vi "sweep_dc.vi"(10 "Cluster 4":T4={"numero di sweep ripetute\n(piramidi per dual sweep)"=3, "Delay Time (S)"=0.001, "Numero di punti"=11, "nplc"=0.1, "dual sweep"=FALSE, "autorange source gate"=FALSE, "source_range_gate"=20.0, "String"="1,2,3", "limit-gate"=1.0, "Source Function Gate"=1, "Range Mode Gate"=0, "range-gate"=0.01, "Autozero Mode Gate"=1, "autorange source drain"=FALSE, "source_range_drain"=2.0, "Pulse Start Level (0 V) 2"=-5.0, "Pulse Stop Level (1 V) 2"=1.0, "limit-drain"=1.0, "Source Function Drain"=1, "Range Mode Drain"=0, "range-drain"=0.01, "Autozero Mode Drain"=1, "inverti smu"=FALSE} {"Autozero Mode Drain" items=["Autozero Off", "Autozero Once", "Autozero Auto"]; "range-drain" items=["100 nA"=1e-07, "1 uA"=1e-06, "10 uA"=1e-05, "100 uA"=0.0001, "1 mA"=0.001, "10 mA"=0.01, "100 mA"=0.1, "1 A"=1.0]; "Range Mode Drain" items=["Auto Range Off", "Auto Range On", "Auto Range Follow Limit"]; "Source Function Drain" items=["Current", "Voltage"]; "limit-drain" format="%#_13g"; "source_range_drain" items=["200 mV"=0.2, "2 V"=2.0, "20 V"=20.0, "200 V"=200.0]; "Autozero Mode Gate" items=["Autozero Off", "Autozero Once", "Autozero Auto"]; "range-gate" items=["100 nA"=1e-07, "1 uA"=1e-06, "10 uA"=1e-05, "100 uA"=0.0001, "1 mA"=0.001, "10 mA"=0.01, "100 mA"=0.1, "1 A"=1.0]; "Range Mode Gate" items=["Auto Range Off", "Auto Range On", "Auto Range Follow Limit"]; "Source Function Gate" items=["Current", "Voltage"]; "limit-gate" format="%#_13g"; "source_range_gate" items=["200 mV"=0.2, "2 V"=2.0, "20 V"=20.0, "200 V"=200.0]; "nplc" items=["0,01"=0.01, "0,1"=0.1, "1"=1.0]}, 11 "Cluster":T3={"VISA resource name"="USB0::0x05E6::0x2612::4671051::INSTR", "error in (no error)"={"status"=FALSE, "code"=0, "source"=""}}) -> (2 "Cluster 3":T1, 3 "Cluster 2":T2)   [LabVIEW 2026]
uses:
  <instrlib>/Keithley 2600 Series/Keithley 2600 Series.lvlib
panel:
  out "range misurato":string
  out "range misurato 2":string
  out "intervallo tra due misure approx (S)":dbl
  out "Frequenza di rete (Hz)":dbl
  out "finestra di misura (S)":dbl
  # "Impostazioni connessione"
  # "tabella valori"
  # "Impostazioni funzione source"
  # "Impostazioni comuni"
  # "DRAIN"
  # "GATE"
  # "non utilizzato...funzioni di lua per automatizzare il range"
  # "Controllo misura"
  # "Impostazioni funzione misura"
  # "DRAIN"
  # "GATE"
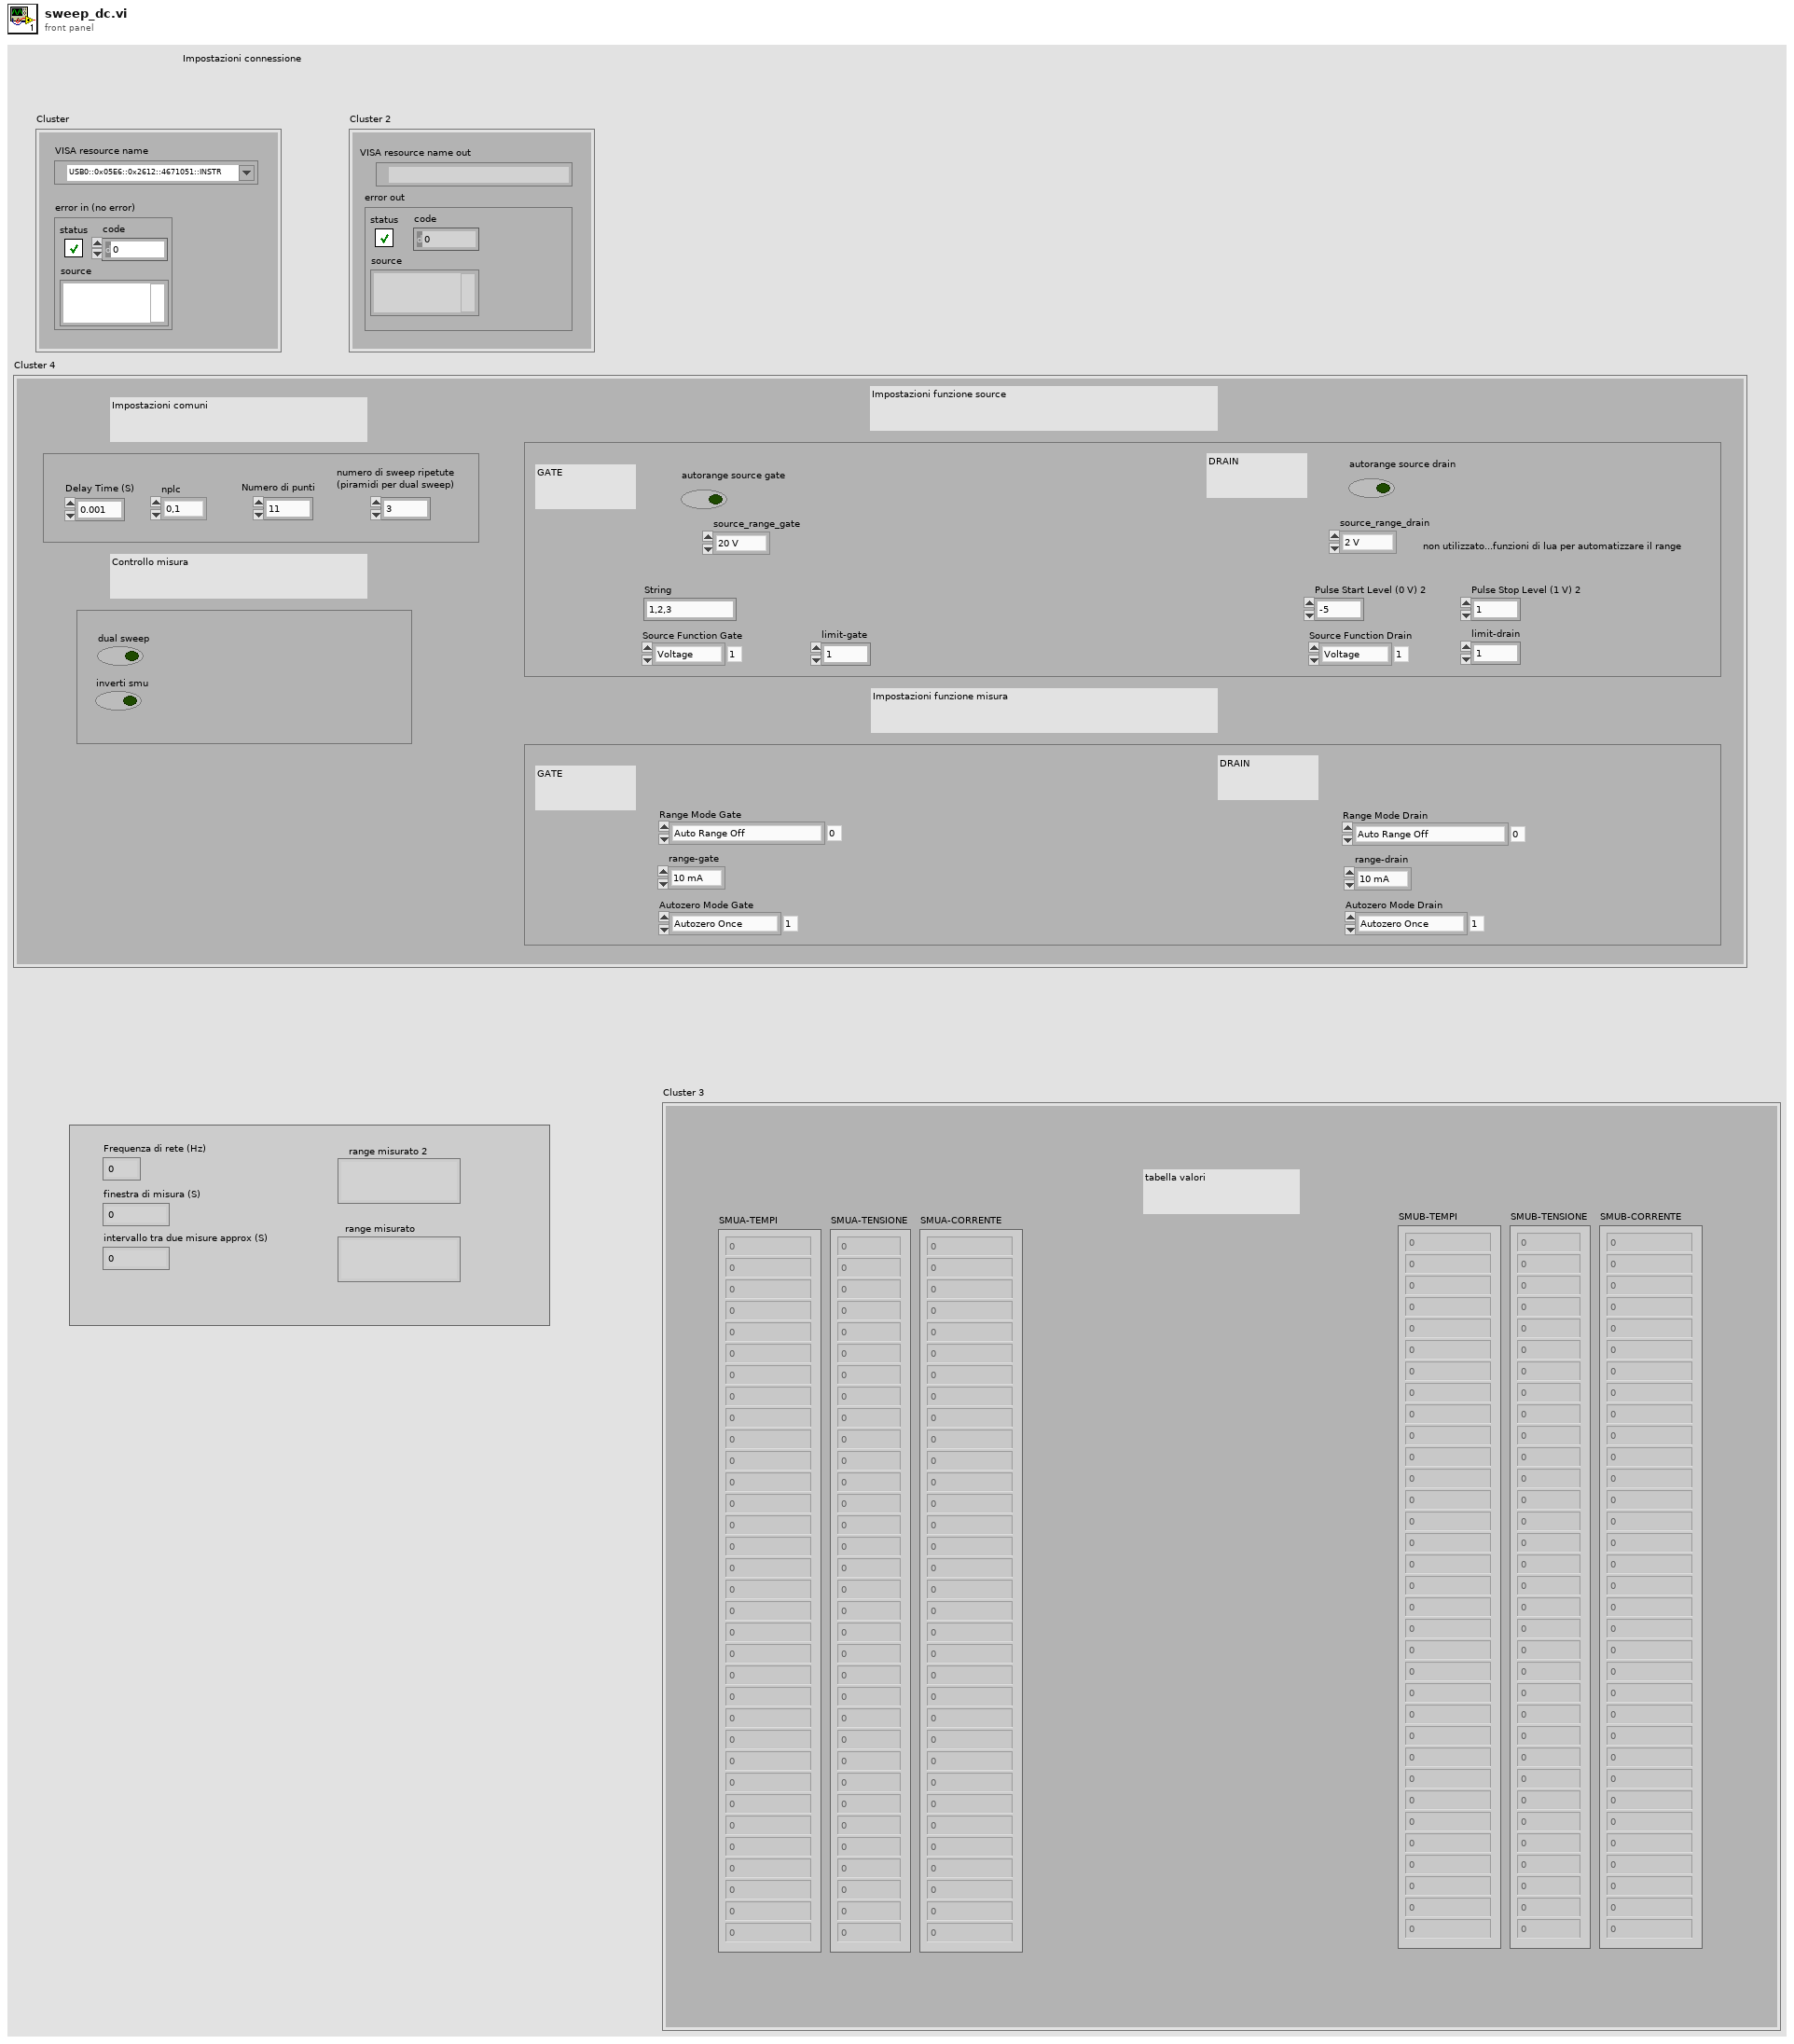
[diagram p1: front panel]
types:
  T1 = cluster{"SMUA-CORRENTE":dbl[], "SMUA-TENSIONE":dbl[], "SMUA-TEMPI":dbl[], "SMUB-CORRENTE":dbl[], "SMUB-TENSIONE":dbl[], "SMUB-TEMPI":dbl[]}
  T2 = cluster{"VISA resource name out":refnum<visa-resource-name>, "error out":errorcluster}
  T3 = cluster{"VISA resource name":refnum<visa-resource-name>, "error in (no error)":errorcluster}
  T4 = cluster{"numero di sweep ripetute\n(piramidi per dual sweep)":i32, "Delay Time (S)":dbl, "Numero di punti":i32, "nplc":dbl, "dual sweep":bool, "autorange source gate":bool, "source_range_gate":dbl, "String":string, "limit-gate":dbl, "Source Function Gate":i32, "Range Mode Gate":i32, "range-gate":dbl, "Autozero Mode Gate":i32, "autorange source drain":bool, "source_range_drain":dbl, "Pulse Start Level (0 V) 2":dbl, "Pulse Stop Level (1 V) 2":dbl, "limit-drain":dbl, "Source Function Drain":i32, "Range Mode Drain":i32, "range-drain":dbl, "Autozero Mode Drain":i32, "inverti smu":bool}
  T5 = cluster{"CORRENTE":dbl[], "TENSIONE":dbl[], "TEMPI":dbl[], "CORRENTE":dbl[], "TENSIONE":dbl[], "TEMPI":dbl[]}
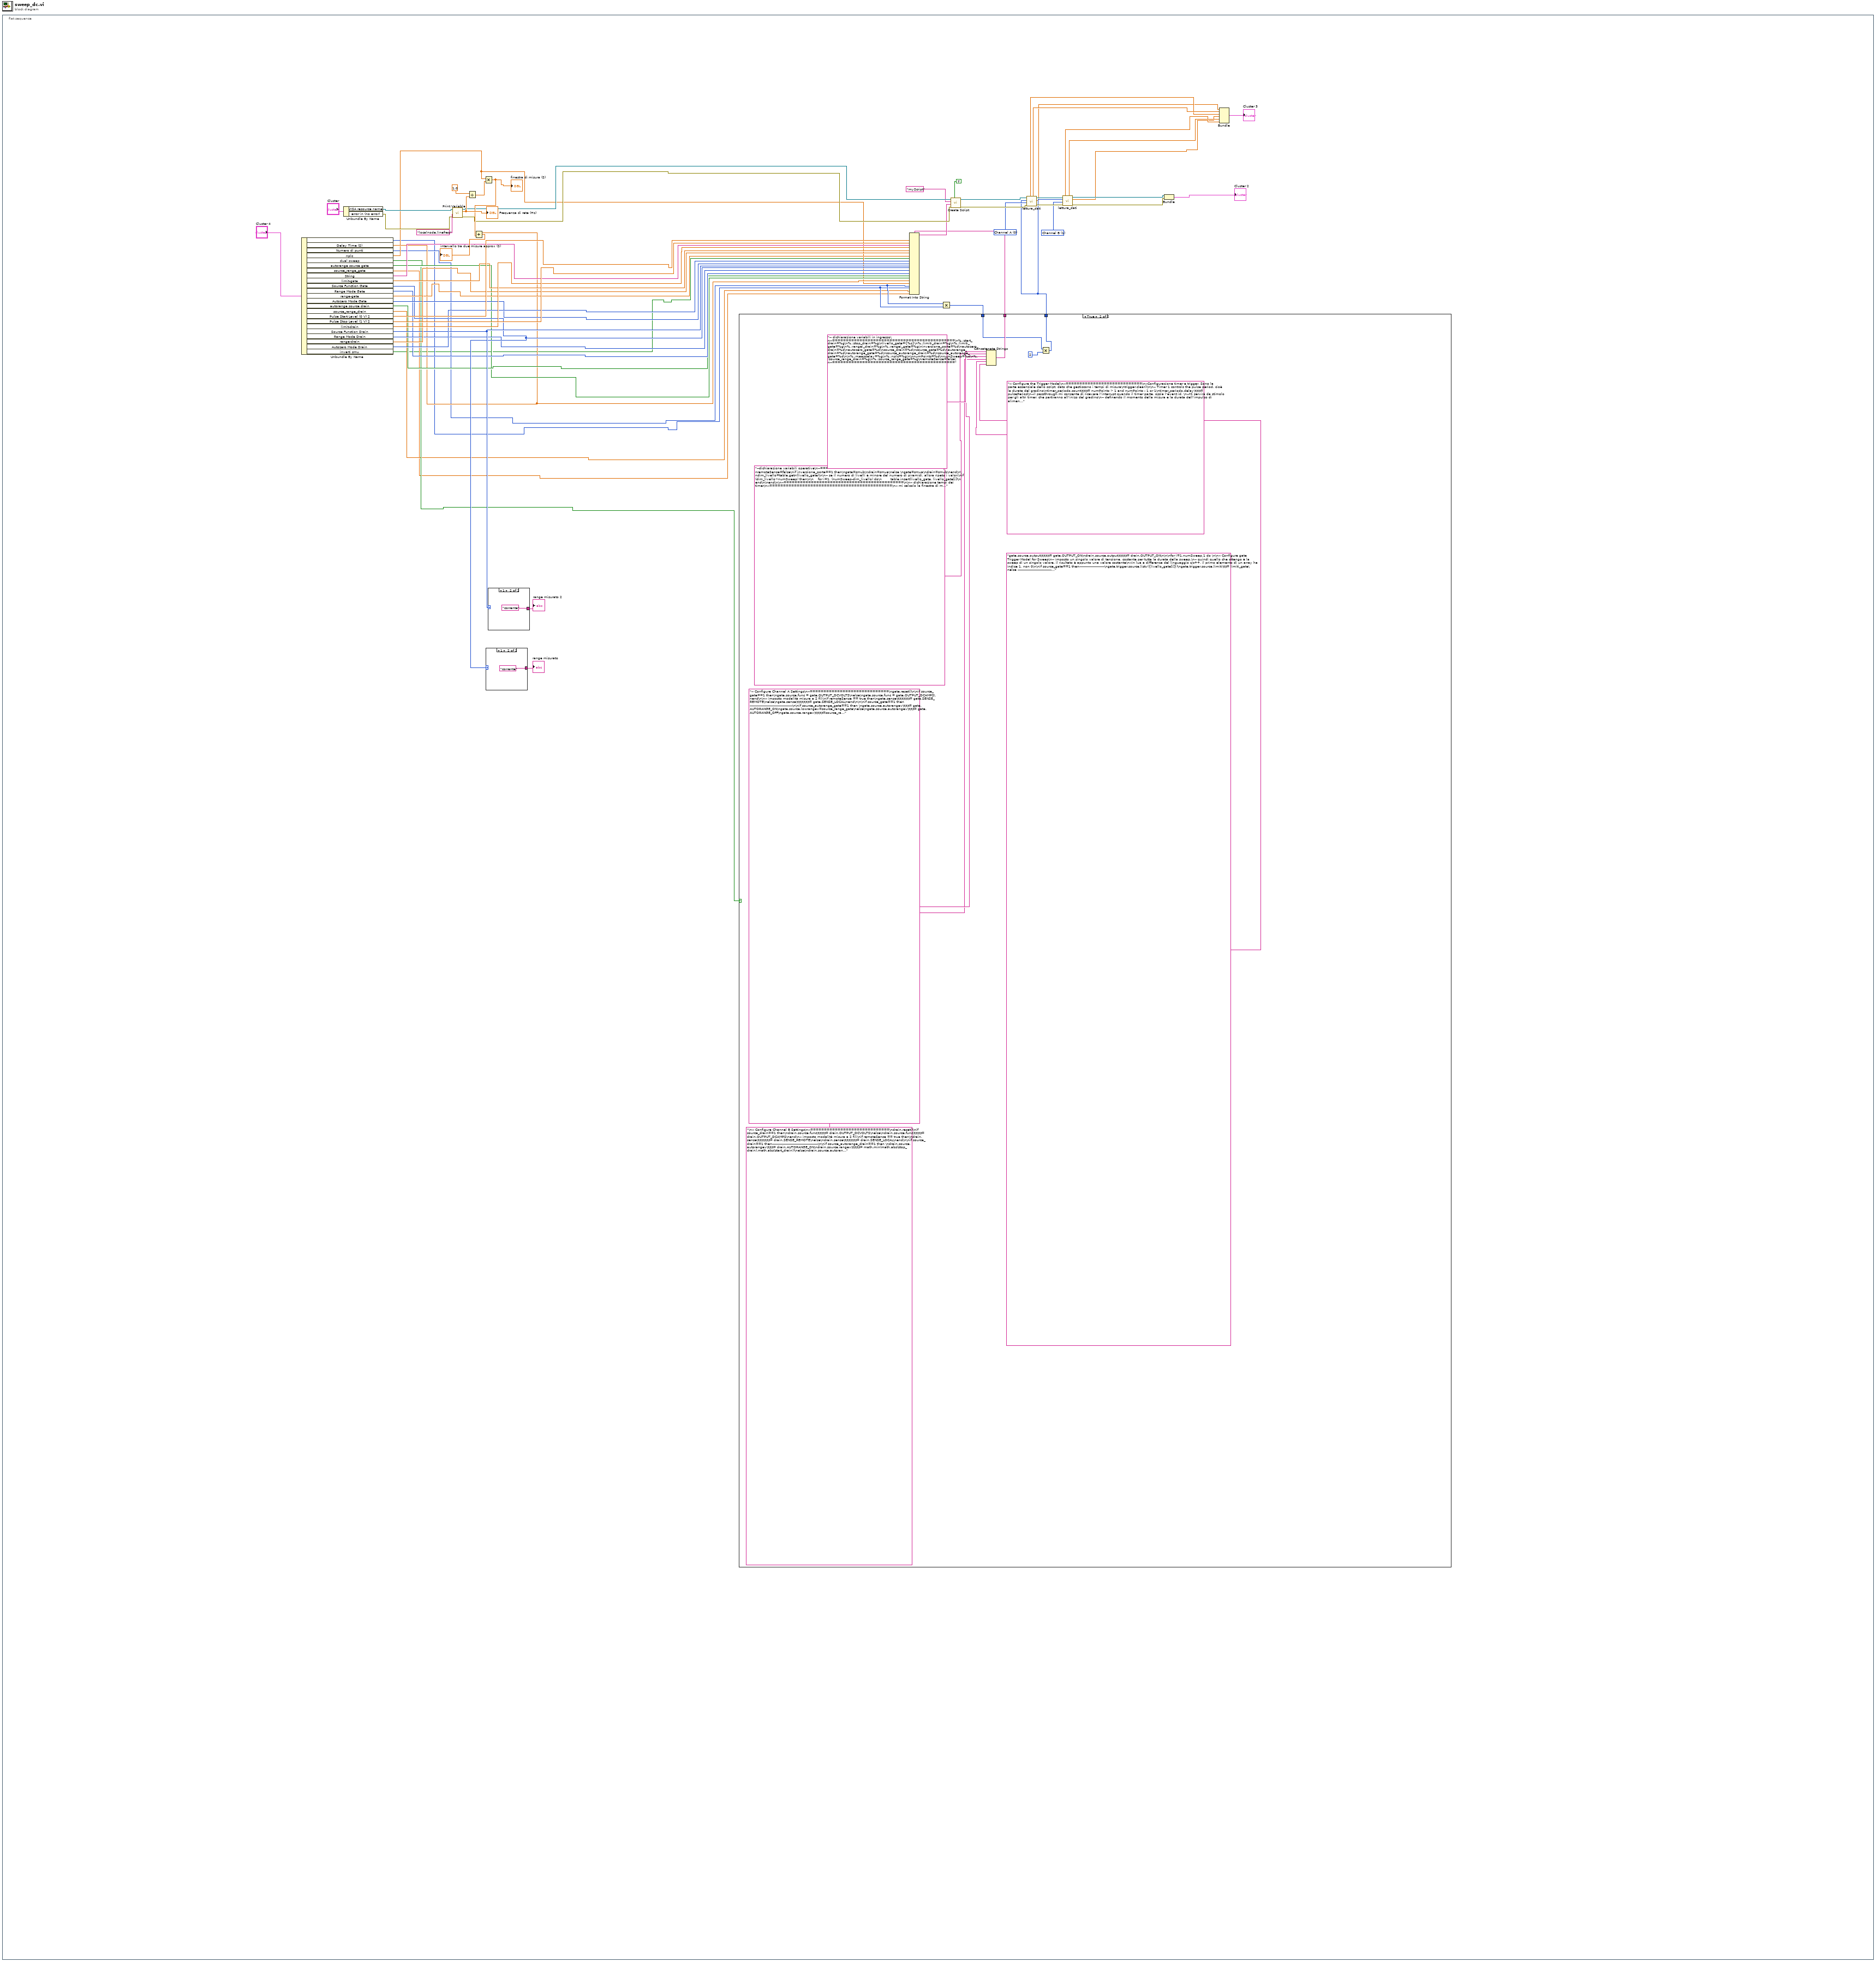
[diagram p0: block diagram]
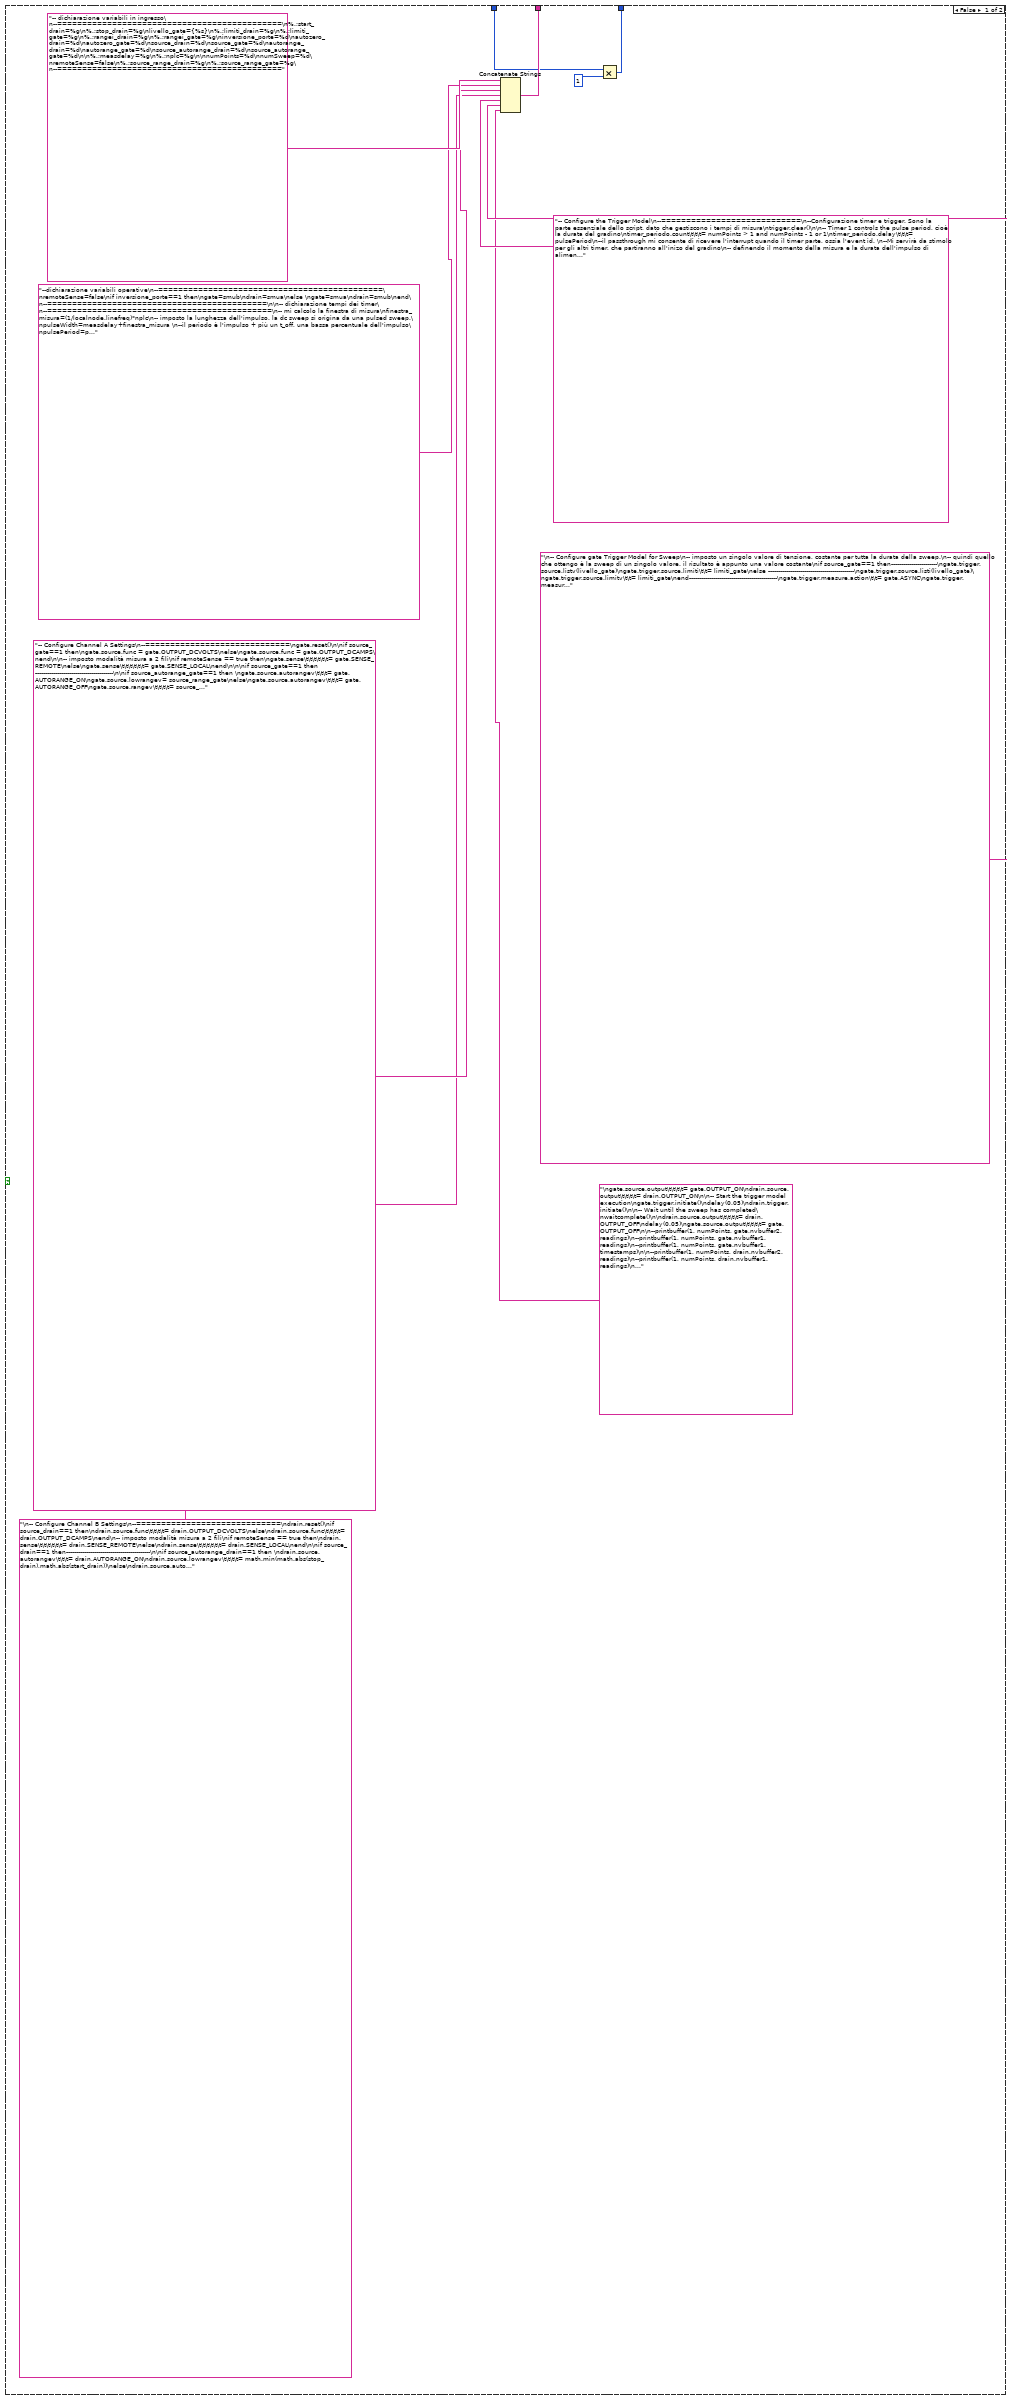
[diagram p2: hidden frame]
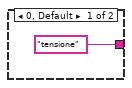
[diagram p3: hidden frame]
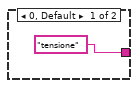
[diagram p4: hidden frame]
diagram:
  n1 = flat-sequence {
    frame #0 {
      w41 = 1 items=["Channel A", "Channel B"] ("Source Measure Unit Channel (0: Channel A)")
      w42 = 0 items=["Channel A", "Channel B"] ("Source Measure Unit Channel (0: Channel A)")
      n2 = Unbundle By Name("Cluster 4") -> ("numero di sweep ripetute\n(piramidi per dual sweep)"=w5:i32, "Delay Time (S)"=w8:dbl, "Numero di punti"=w6:i32, "nplc"=w7:dbl, "dual sweep"=w4:bool, "autorange source gate"=w9:bool, "source_range_gate"=w2:dbl, "String"=w21:string, "limit-gate"=w19:dbl, "Source Function Gate"=w13:i32, "Range Mode Gate"=w11:i32, "range-gate"=w17:dbl, "Autozero Mode Gate"=w15:i32, "autorange source drain"=w10:bool, "source_range_drain"=w3:dbl, "Pulse Start Level (0 V) 2"=w23:dbl, "Pulse Stop Level (1 V) 2"=w22:dbl, "limit-drain"=w20:dbl, "Source Function Drain"=w14:i32, "Range Mode Drain"=w12:i32, "range-drain"=w18:dbl, "Autozero Mode Drain"=w16:i32, "inverti smu"=w1:bool)
      n3 = Unbundle By Name("Cluster") -> ("VISA resource name"=w31:refnum<visa-resource-name>, "error in (no error)"=w30:errorcluster)
      n4 = call <instrlib>:"Print Variable.vi"("error in (no error)"=w30, "Variable Name"="localnode.linefreq", "VISA resource name"=w31) -> ("error out"=w52:errorcluster, "Number"=w56:dbl, "VISA resource name out"=w53:refnum<visa-resource-name>)  [unwired: 5 in, 1 out]
      "Frequenza di rete (Hz)" <- w56
      n5 = Divide(x=1.0, y=w56) -> (x/y=w58:dbl)
      n6 = Multiply(x=w7, y=w58) -> (x*y=w54:dbl)
      "finestra di misura (S)" <- w54
      n7 = Add(x=w8, y=w54) -> (x+y=→"intervallo tra due misure approx (S)":dbl)
      n8 = case shown="1" w13 {
        tunnel: ["tensione" "corrente"] -> w50
        frame 0, Default {
        }
        frame 1 {
        }
      }
      "range misurato" <- w50
      n9 = case shown="1" w14 {
        tunnel: ["tensione" "corrente"] -> w51
        frame 0, Default {
        }
        frame 1 {
        }
      }
      "range misurato 2" <- w51
      n10 = Multiply(x=w6, y=w5) -> (x*y=w39:i32)
      n11 = case shown="True" w4 {
        tunnel: [w63 w74] -> w40
        tunnel: w39 -> [w62 w72]
        tunnel: [w61 w73] -> w38
        frame False {
          n12 = Concatenate Strings("-- dichiarazione variabili in ingresso\n--=============================================\n%.;start_drain=%g\n%.;stop_drain=%g\nlivello_gate={%s}\n%.;limiti_drain=%g\n%.;limiti_gate=%g\n%.;rangei_drain=%g\n%.;rangei_gate=%g\ninversione_porte=%d\nautozero_drain=%d\nautozero_gate=%d\nsource_drain=%d\nsource_gate=%d\nautorange_drain=%d\nautorange_gate=%d\nsource_autorange_drain=%d\nsource_autorange_gate=%d\n\n%.;measdelay=%g\n%.;nplc=%g\n\nnumPoints=%d\nnumSweep=%d\nremoteSense=false\n%.;source_range_drain=%g\n%.;source_range_gate=%g\n--=============================================", "--dichiarazione variabili operative\n--=============================================\nremoteSense=false\nif inversione_porte==1 then\ngate=smub\ndrain=smua\nelse \ngate=smua\ndrain=smub\nend\n--============================================\n\n-- dichiarazione tempi dei timer\n--=============================================\n-- mi calcolo la finestra di misura\nfinestra_misura=(1/localnode.linefreq)*nplc\n-- imposto la lunghezza dell'impulso. la dc sweep si origina da una pulsed sweep.\npulseWidth=measdelay+finestra_misura \n--il periodo è l'impulso + più un t_off, una bassa percentuale dell'impulso\npulsePeriod=pulseWidth+(pulseWidth*1/100) \n\n--=============================================\n\n-- dichiarazione timer e gestore eventi\n--=============================================\n-- Timer 1: timer periodo (larghezza gradino)\ntimer_periodo=trigger.timer[1]\n-- Timer 2: Timer ritardo misura\ntimer_misura=trigger.timer[2]\n-- Timer 3: Pulse Width Timer\ntimer_larghezza_impulso=trigger.timer[3]\n\n-- Gestore eventi 1: Event Blender per la partenza di iniziale di smua e l'aggiornamento di smua al trigger di smub\ngestore_avvio_gate=trigger.blender[1]\n--=============================================", "-- Configure Channel A Settings\n--=============================\ngate.reset()\n\nif source_gate==1 then\ngate.source.func = gate.OUTPUT_DCVOLTS\nelse\ngate.source.func = gate.OUTPUT_DCAMPS\nend\n\n-- imposto modalità misura a 2 fili\nif remoteSense == true then\ngate.sense\t\t\t\t\t\t= gate.SENSE_REMOTE\nelse\ngate.sense\t\t\t\t\t\t= gate.SENSE_LOCAL\nend\n\n\nif source_gate==1 then ---------------------------------------\n\nif source_autorange_gate==1 then \ngate.source.autorangev\t\t\t= gate.AUTORANGE_ON\ngate.source.lowrangev= source_range_gate\nelse\ngate.source.autorangev\t\t\t= gate.AUTORANGE_OFF\ngate.source.rangev\t\t\t\t= source_range_gate\nend \n\ngate.source.levelv\t\t\t\t= 0\n-- Set the DC bias limit.  This is not the limit used during the pulses. ma è il valore di idle della gate\ngate.source.limiti\t\t\t\t= limiti_gate\n\nelse------------------------\n\nif source_autorange_gate==1 then\ngate.source.autorangei\t\t\t= gate.AUTORANGE_ON\ngate.source.lowrangei=source_range_gate\nelse\ngate.source.autorangei\t\t\t= gate.AUTORANGE_OFF\ngate.source.rangei\t\t\t=source_range_gate\nend\n\ngate.source.leveli\t\t\t\t= 0\n-- Set the DC bias limit.  This is not the limit used during the pulses. ma è il valore di idle della gate\ngate.source.limitv\t\t\t\t= limiti_gate\nend --------------------------------------------------\n\n\n-- Disabling Auto-Ranging and Auto-Zero ensures accurate and consistent timing\nif autozero_gate==0 then\ngate.measure.autozero\t\t\t= gate.AUTOZERO_OFF\nelseif autozero_gate==1 then\ngate.measure.autozero\t\t\t= gate.AUTOZERO_ONCE\nelse\ngate.measure.autozero\t\t\t= gate.AUTOZERO_AUTO\nend\n\nif autorange_gate==0 then ------------------------\n\nif source_gate==1 then\ngate.measure.autorangei\t\t\t= gate.AUTORANGE_OFF\ngate.measure.rangei\t\t\t\t= rangei_gate\nelse\ngate.measure.autorangev\t\t\t= gate.AUTORANGE_OFF\ngate.measure.rangev\t\t\t\t= rangei_gate\nend\n\nelseif  autorange_gate==1 then -----------\n\nif source_gate==1 then\ngate.measure.autorangei\t\t\t= gate.AUTORANGE_ON\ngate.measure.lowrangei\t\t\t\t= rangei_gate\nelse\ngate.measure.autorangev\t\t\t= gate.AUTORANGE_ON\ngate.measure.lowrangev\t\t\t\t= rangei_gate\nend\n\nelse --------------------------\n\nend -------------------------------\n\ngate.measure.nplc\t\t\t\t= nplc\n-- A timer will be used to set the measure delay and synchronize the measurement\n-- between the two SMUs so set the built in delay to 0.\ngate.measure.delay\t\t\t\t= 0\n\n-- Prepare the Reading Buffers\ngate.nvbuffer1.clear()\ngate.nvbuffer1.collecttimestamps= 1\ngate.nvbuffer2.clear()\ngate.nvbuffer2.collecttimestamps = 1\n--=============================\n-- End Channel A Settings", "\n-- Configure Channel B Settings\n--=============================\ndrain.reset()\nif source_drain==1 then\ndrain.source.func\t\t\t\t= drain.OUTPUT_DCVOLTS\nelse\ndrain.source.func\t\t\t\t= drain.OUTPUT_DCAMPS\nend\n-- imposto modalità misura a 2 fili\nif remoteSense == true then\ndrain.sense\t\t\t\t\t\t= drain.SENSE_REMOTE\nelse\ndrain.sense\t\t\t\t\t\t= drain.SENSE_LOCAL\nend\n\nif source_drain==1 then------------------------------------------\n\nif source_autorange_drain==1 then \ndrain.source.autorangev\t\t\t= drain.AUTORANGE_ON\ndrain.source.lowrangev\t\t\t\t= math.min(math.abs(stop_drain),math.abs(start_drain))\nelse\ndrain.source.autorangev\t\t\t= drain.AUTORANGE_OFF\ndrain.source.rangev\t\t\t\t=  math.max(math.abs(stop_drain),math.abs(start_drain))\nend\n\ndrain.source.levelv\t\t\t\t= 0\n-- Set the DC bias limit.  This is not the limit used during the pulses. ma è il valore di idle della smu\ndrain.source.limiti\t\t\t\t= limiti_drain\nelse----------------------------------------------------\nif source_autorange_drain==1 then \ndrain.source.autorangei\t\t\t= drain.AUTORANGE_ON\ndrain.source.lowrangei\t\t\t\t= math.min(math.abs(stop_drain),math.abs(start_drain))\nelse\ndrain.source.autorangei\t\t\t= drain.AUTORANGE_OFF\ndrain.source.rangei\t\t\t\t= math.max(math.abs(stop_drain),math.abs(start_drain))\nend\ndrain.source.leveli\t\t\t\t= 0\n-- Set the DC bias limit.  This is not the limit used during the pulses. ma è il valore di idle della smu\ndrain.source.limitv\t\t\t\t= limiti_drain\nend----------------------------------------------\n\n-- Disabling Auto-Ranging and Auto-Zero ensures accurate and consistent timing\n\nif autozero_drain==0 then\ndrain.measure.autozero\t\t\t= drain.AUTOZERO_OFF\nelseif autozero_drain==1 then\ndrain.measure.autozero\t\t\t= drain.AUTOZERO_ONCE\nelseif autozero_drain==2 then\ndrain.measure.autozero\t\t\t= drain.AUTOZERO_AUTO\nend\n\nif autorange_drain==0 then --------------------------------\n\nif source_drain==1 then\ndrain.measure.autorangei\t\t\t= drain.AUTORANGE_OFF\ndrain.measure.rangei\t\t\t\t= rangei_drain\nelse\ndrain.measure.autorangev\t\t\t= drain.AUTORANGE_OFF\ndrain.measure.rangev\t\t\t\t= rangei_drain\nend\n\n\n\nelseif  autorange_drain==1 then ----------------------------\n\nif source_drain==1 then\ndrain.measure.autorangei\t\t\t= drain.AUTORANGE_ON\ndrain.measure.lowrangei\t\t\t\t= rangei_drain\nelse\ndrain.measure.autorangev\t\t\t= drain.AUTORANGE_ON\ndrain.measure.lowrangev\t\t\t\t= rangei_drain\nend\n\nelse\n\nend --------------------------------------------------------------\n\ndrain.measure.nplc\t\t\t\t= nplc\n-- A timer will be used to set the measure delay and synchronize the measurement\n-- between the two SMUs so set the built in delay to 0.\ndrain.measure.delay\t\t\t\t= 0\n\n-- Prepare the Reading Buffers\ndrain.nvbuffer1.clear()\ndrain.nvbuffer1.collecttimestamps= 1\ndrain.nvbuffer2.clear()\ndrain.nvbuffer2.collecttimestamps= 1\n--=============================\n-- End Channel B Settings", "-- Configure the Trigger Model\n--============================\n--Configurazione timer e trigger. Sono la parte essenziale dello script, dato che gestiscono i tempi di misura\ntrigger.clear()\n\n-- Timer 1 controls the pulse period, cioè la durata del gradino\ntimer_periodo.count\t\t\t= numPoints > 1 and numPoints - 1 or 1\ntimer_periodo.delay\t\t\t= pulsePeriod\n--il passthrough mi consente di ricevere l'interrupt quando il timer parte, ossia l'event id. \n--Mi servirà da stimolo per gli altri timer, che partiranno all'inizo del gradino\n-- definendo il momento della misura e la durata dell'impulso di alimentazione\ntimer_periodo.passthrough\t= true\n-- il timer 1 parte quando la drain, in questo caso, inizia la sweep: cioè entra nello stato armed\ntimer_periodo.stimulus\t\t= drain.trigger.ARMED_EVENT_ID \n\n-- Timer 2 controls the measurement. il timer 2 gestisce il ritardo di misura. scaduto quello, inizia la finestra di misura\ntimer_misura.count\t\t\t= 1\ntimer_misura.delay\t\t\t= measdelay\n-- il passthrough è false perchè l'interrupt lo produrre alla fine. \n-- Scaduto il delay di misura, inizia la finestra di misura\ntimer_misura.passthrough\t= false\n--il timer 1 grazie al passthrough mi fa partire il timer 2 all'inizio del gradino\ntimer_misura.stimulus\t\t= timer_periodo.EVENT_ID \n\n-- Timer 3 controls the pulse width\ntimer_larghezza_impulso.count\t\t\t= 1\ntimer_larghezza_impulso.delay\t\t\t= pulseWidth\n-- il passthrough è false perchè l'interrupt me lo produce alla fine, perchè \ntimer_larghezza_impulso.passthrough\t= false\n--il timer 1 grazie al passthrough mi fa partire il timer 3 all'inizio del gradino\ntimer_larghezza_impulso.stimulus\t\t= timer_periodo.EVENT_ID\n", "\n-- Configure gate Trigger Model for Sweep\n-- imposto un singolo valore di tensione, costante per tutta la durata della sweep.\n-- quindi quello che ottengo è la sweep di un singolo valore. il risultato è appunto una valore costante\nif source_gate==1 then-----------------------\ngate.trigger.source.listv(livello_gate)\ngate.trigger.source.limiti\t\t= limiti_gate\nelse -------------------------------------------\ngate.trigger.source.listi(livello_gate)\ngate.trigger.source.limitv\t\t= limiti_gate\nend--------------------------------------------\ngate.trigger.measure.action\t\t= gate.ASYNC\ngate.trigger.measure.iv(gate.nvbuffer1, gate.nvbuffer2)\n--fine impulso: se voglio una dc sweep, anzichè mandare in idle l'uscita, la tengo costante\ngate.trigger.endpulse.action\t= gate.SOURCE_HOLD\n-- endsweep mi dice cosa fare quando finisce l'operazione sweep\ngate.trigger.endsweep.action\t= gate.SOURCE_HOLD\ngate.trigger.arm.count = 1\ngate.trigger.count\t\t\t\t= numSweep\n-- arm sweep indica quanto sweep deve fare \ndrain.trigger.arm.stimulus\t\t= 0\n\n\n--event blender per la partenza\ngestore_avvio_gate.orenable = true\ngestore_avvio_gate.stimulus[1] = gate.trigger.ARMED_EVENT_ID\ngestore_avvio_gate.stimulus[2] = drain.trigger.ARMED_EVENT_ID \n\n--dico quali stimoli/timer attivano le azioni\ngate.trigger.source.stimulus = gestore_avvio_gate.EVENT_ID \ngate.trigger.measure.stimulus\t= timer_misura.EVENT_ID\ngate.trigger.endpulse.stimulus\t= drain.trigger.SWEEP_COMPLETE_EVENT_ID\n\ngate.trigger.source.action\t\t= gate.ENABLE\n\n-- Configure drain Trigger Model for Sweep\nif source_drain==1 then------------------------\ndrain.trigger.source.linearv(start_drain, stop_drain, numPoints)\ndrain.trigger.source.limiti\t\t= limiti_drain\nelse---------------------------------------------\ndrain.trigger.source.lineari(start_drain, stop_drain, numPoints)\ndrain.trigger.source.limitv\t\t= limiti_drain\nend---------------------------------------------\ndrain.trigger.measure.action\t\t= drain.ENABLE\ndrain.trigger.measure.iv(drain.nvbuffer1, drain.nvbuffer2)\n--fine impulso: se voglio una dc sweep, anzichè mandare in idle l'uscita, la tengo costante\ndrain.trigger.endpulse.action\t= drain.SOURCE_HOLD \n-- endsweep mi dice cosa fare quando finisce l'operazione sweep\ndrain.trigger.endsweep.action\t= drain.SOURCE_HOLD\ndrain.trigger.arm.count = numSweep\n-- num punti sweep\ndrain.trigger.count\t\t\t\t= numPoints\n-- arm sweep indica quanto sweep deve fare\ndrain.trigger.arm.stimulus\t\t= 0\n--dico quali timer attivanzo le azioni\ndrain.trigger.source.stimulus\t= timer_periodo.EVENT_ID\ndrain.trigger.measure.stimulus\t= timer_misura.EVENT_ID\ndrain.trigger.endpulse.stimulus\t= timer_larghezza_impulso.EVENT_ID\ndrain.trigger.source.action\t\t= drain.ENABLE\n--==============================\n-- End Trigger Model Configuration" ("write buffer"), "\ngate.source.output\t\t\t\t= gate.OUTPUT_ON\ndrain.source.output\t\t\t\t= drain.OUTPUT_ON\n\n-- Start the trigger model execution\ngate.trigger.initiate()\ndelay(0.05)\ndrain.trigger.initiate()\n\n-- Wait until the sweep has completed\nwaitcomplete()\n\ndrain.source.output\t\t\t\t= drain.OUTPUT_OFF\ndelay(0.05)\ngate.source.output\t\t\t\t= gate.OUTPUT_OFF\n\n--printbuffer(1, numPoints, gate.nvbuffer2.readings)\n--printbuffer(1, numPoints, gate.nvbuffer1.readings)\n--printbuffer(1, numPoints, gate.nvbuffer1.timestamps)\n\n--printbuffer(1, numPoints, drain.nvbuffer2.readings)\n--printbuffer(1, numPoints, drain.nvbuffer1.readings)\n--printbuffer(1, numPoints, drain.nvbuffer1.timestamps)\n") -> (w63:string)
          n13 = Multiply(x=w62, y=1) -> (x*y=w61:i32)
        }
        frame True {
          n14 = Concatenate Strings("-- dichiarazione variabili in ingresso\n--=============================================\n%.;start_drain=%g\n%.;stop_drain=%g\nlivello_gate={%s}\n%.;limiti_drain=%g\n%.;limiti_gate=%g\n%.;rangei_drain=%g\n%.;rangei_gate=%g\ninversione_porte=%d\nautozero_drain=%d\nautozero_gate=%d\nsource_drain=%d\nsource_gate=%d\nautorange_drain=%d\nautorange_gate=%d\nsource_autorange_drain=%d\nsource_autorange_gate=%d\n\n%.;measdelay=%g\n%.;nplc=%g\n\nnumPoints=%d\nnumSweep=%d\n%.;source_range_drain=%g\n%.;source_range_gate=%g\nremoteSense=false\n--=============================================", "--dichiarazione variabili operative\n--=============================================\nremoteSense=false\nif inversione_porte==1 then\ngate=smub\ndrain=smua\nelse \ngate=smua\ndrain=smub\nend\n\ndim_livello=table.getn(livello_gate)\n\n-- se il numero di livelli è minore del numero di piramidi, allora ripeto i valori\nif (dim_livello<numSweep) then\n\n    for i=1, (numSweep-dim_livello) do\n        table.insert(livello_gate, livello_gate[i])\n    end\n\nend\n\n--============================================\n\n-- dichiarazione tempi dei timer\n--=============================================\n-- mi calcolo la finestra di misura\nfinestra_misura=(1/localnode.linefreq)*nplc\n-- imposto la lunghezza dell'impulso. la dc sweep si origina da una pulsed sweep.\npulseWidth=measdelay+finestra_misura \n--il periodo è l'impulso + più un t_off, una bassa percentuale dell'impulso\npulsePeriod=pulseWidth+(pulseWidth*1/100) \n--=============================================\n\n-- dichiarazione timer e gestore eventi\n--=============================================\n-- Timer 1: timer periodo (larghezza gradino)\ntimer_periodo=trigger.timer[1]\n-- Timer 2: Timer ritardo misura\ntimer_misura=trigger.timer[2]\n-- Timer 3: Pulse Width Timer\ntimer_larghezza_impulso=trigger.timer[3]\n\n-- Gestore eventi 1: Event Blender per la partenza di iniziale di smua e l'aggiornamento di smua al trigger di smub\ngestore_avvio_gate=trigger.blender[1]\n--=============================================", "-- Configure Channel A Settings\n--=============================\ngate.reset()\n\nif source_gate==1 then\ngate.source.func = gate.OUTPUT_DCVOLTS\nelse\ngate.source.func = gate.OUTPUT_DCAMPS\nend\n\n-- imposto modalità misura a 2 fili\nif remoteSense == true then\ngate.sense\t\t\t\t\t\t= gate.SENSE_REMOTE\nelse\ngate.sense\t\t\t\t\t\t= gate.SENSE_LOCAL\nend\n\n\nif source_gate==1 then ---------------------------------------\n\nif source_autorange_gate==1 then \ngate.source.autorangev\t\t\t= gate.AUTORANGE_ON\ngate.source.lowrangev=source_range_gate\nelse\ngate.source.autorangev\t\t\t= gate.AUTORANGE_OFF\ngate.source.rangev\t\t\t\t=source_range_gate\nend \n\ngate.source.levelv\t\t\t\t= 0\n-- Set the DC bias limit.  This is not the limit used during the pulses. ma è il valore di idle della gate\ngate.source.limiti\t\t\t\t= limiti_gate\n\nelse------------------------\n\nif source_autorange_gate==1 then\ngate.source.autorangei\t\t\t= gate.AUTORANGE_ON\ngate.source.lowrangei=source_range_gate\nelse\ngate.source.autorangei\t\t\t= gate.AUTORANGE_OFF\ngate.source.rangei\t\t\t=source_range_gate\nend\n\ngate.source.leveli\t\t\t\t= 0\n-- Set the DC bias limit.  This is not the limit used during the pulses. ma è il valore di idle della gate\ngate.source.limitv\t\t\t\t= limiti_gate\nend --------------------------------------------------\n\n\n-- Disabling Auto-Ranging and Auto-Zero ensures accurate and consistent timing\nif autozero_gate==0 then\ngate.measure.autozero\t\t\t= gate.AUTOZERO_OFF\nelseif autozero_gate==1 then\ngate.measure.autozero\t\t\t= gate.AUTOZERO_ONCE\nelse\ngate.measure.autozero\t\t\t= gate.AUTOZERO_AUTO\nend\n\nif autorange_gate==0 then ------------------------\n\nif source_gate==1 then\ngate.measure.autorangei\t\t\t= gate.AUTORANGE_OFF\ngate.measure.rangei\t\t\t\t= rangei_gate\nelse\ngate.measure.autorangev\t\t\t= gate.AUTORANGE_OFF\ngate.measure.rangev\t\t\t\t= rangei_gate\nend\n\nelseif  autorange_gate==1 then -----------\n\nif source_gate==1 then\ngate.measure.autorangei\t\t\t= gate.AUTORANGE_ON\ngate.measure.lowrangei\t\t\t\t= rangei_gate\nelse\ngate.measure.autorangev\t\t\t= gate.AUTORANGE_ON\ngate.measure.lowrangev\t\t\t\t= rangei_gate\nend\n\nelse --------------------------\n\nend -------------------------------\n\ngate.measure.nplc\t\t\t\t= nplc\n-- A timer will be used to set the measure delay and synchronize the measurement\n-- between the two SMUs so set the built in delay to 0.\ngate.measure.delay\t\t\t\t= 0\n\n-- Prepare the Reading Buffers\ngate.nvbuffer1.clear()\ngate.nvbuffer1.collecttimestamps= 1\ngate.nvbuffer1.appendmode=1\ngate.nvbuffer2.clear()\ngate.nvbuffer2.collecttimestamps = 1\ngate.nvbuffer2.appendmode=1\n--=============================\n-- End Channel A Settings", "\n-- Configure Channel B Settings\n--=============================\ndrain.reset()\nif source_drain==1 then\ndrain.source.func\t\t\t\t= drain.OUTPUT_DCVOLTS\nelse\ndrain.source.func\t\t\t\t= drain.OUTPUT_DCAMPS\nend\n-- imposto modalità misura a 2 fili\nif remoteSense == true then\ndrain.sense\t\t\t\t\t\t= drain.SENSE_REMOTE\nelse\ndrain.sense\t\t\t\t\t\t= drain.SENSE_LOCAL\nend\n\nif source_drain==1 then------------------------------------------\n\nif source_autorange_drain==1 then \ndrain.source.autorangev\t\t\t= drain.AUTORANGE_ON\ndrain.source.rangev\t\t\t\t= math.min(math.abs(stop_drain),math.abs(start_drain))\nelse\ndrain.source.autorangev\t\t\t= drain.AUTORANGE_OFF\ndrain.source.rangev\t\t\t\t=  math.max(math.abs(stop_drain),math.abs(start_drain))\nend\n\ndrain.source.levelv\t\t\t\t= 0\n-- Set the DC bias limit.  This is not the limit used during the pulses. ma è il valore di idle della smu\ndrain.source.limiti\t\t\t\t= limiti_drain\nelse----------------------------------------------------\nif source_autorange_drain==1 then \ndrain.source.autorangei\t\t\t= drain.AUTORANGE_ON\ndrain.source.rangei\t\t\t\t= math.min(math.abs(stop_drain),math.abs(start_drain))\nelse\ndrain.source.autorangei\t\t\t= drain.AUTORANGE_OFF\ndrain.source.rangei\t\t\t\t= math.max(math.abs(stop_drain),math.abs(start_drain))\nend\ndrain.source.leveli\t\t\t\t= 0\n-- Set the DC bias limit.  This is not the limit used during the pulses. ma è il valore di idle della smu\ndrain.source.limitv\t\t\t\t= limiti_drain\nend----------------------------------------------\n\n-- Disabling Auto-Ranging and Auto-Zero ensures accurate and consistent timing\n\nif autozero_drain==0 then\ndrain.measure.autozero\t\t\t= drain.AUTOZERO_OFF\nelseif autozero_drain==1 then\ndrain.measure.autozero\t\t\t= drain.AUTOZERO_ONCE\nelseif autozero_drain==2 then\ndrain.measure.autozero\t\t\t= drain.AUTOZERO_AUTO\nend\n\nif autorange_drain==0 then --------------------------------\n\nif source_drain==1 then\ndrain.measure.autorangei\t\t\t= drain.AUTORANGE_OFF\ndrain.measure.rangei\t\t\t\t= rangei_drain\nelse\ndrain.measure.autorangev\t\t\t= drain.AUTORANGE_OFF\ndrain.measure.rangev\t\t\t\t= rangei_drain\nend\n\n\n\nelseif  autorange_drain==1 then ----------------------------\n\nif source_drain==1 then\ndrain.measure.autorangei\t\t\t= drain.AUTORANGE_ON\ndrain.measure.lowrangei\t\t\t\t= rangei_drain\nelse\ndrain.measure.autorangev\t\t\t= drain.AUTORANGE_ON\ndrain.measure.lowrangev\t\t\t\t= rangei_drain\nend\n\nelse\n\nend --------------------------------------------------------------\n\ndrain.measure.nplc\t\t\t\t= nplc\n-- A timer will be used to set the measure delay and synchronize the measurement\n-- between the two SMUs so set the built in delay to 0.\ndrain.measure.delay\t\t\t\t= 0\n\n-- Prepare the Reading Buffers\ndrain.nvbuffer1.clear()\ndrain.nvbuffer1.collecttimestamps= 1\ndrain.nvbuffer1.appendmode=1\ndrain.nvbuffer2.clear()\ndrain.nvbuffer2.collecttimestamps= 1\ndrain.nvbuffer2.appendmode=1\n--=============================\n-- End Channel B Settings", "-- Configure the Trigger Model\n--============================\n--Configurazione timer e trigger. Sono la parte essenziale dello script, dato che gestiscono i tempi di misura\ntrigger.clear()\n\n-- Timer 1 controls the pulse period, cioè la durata del gradino\ntimer_periodo.count\t\t\t= numPoints > 1 and numPoints - 1 or 1\ntimer_periodo.delay\t\t\t= pulsePeriod\n--il passthrough mi consente di ricevere l'interrupt quando il timer parte, ossia l'event id. \n--Mi servirà da stimolo per gli altri timer, che partiranno all'inizo del gradino\n-- definendo il momento della misura e la durata dell'impulso di alimentazione\ntimer_periodo.passthrough\t= true\n-- il timer 1 parte quando la drain, in questo caso, inizia la sweep: cioè entra nello stato armed\ntimer_periodo.stimulus\t\t= drain.trigger.ARMED_EVENT_ID \n\n-- Timer 2 controls the measurement. il timer 2 gestisce il ritardo di misura. scaduto quello, inizia la finestra di misura\ntimer_misura.count\t\t\t= 1\ntimer_misura.delay\t\t\t= measdelay\n-- il passthrough è false perchè l'interrupt lo produrre alla fine. \n-- Scaduto il delay di misura, inizia la finestra di misura\ntimer_misura.passthrough\t= false\n--il timer 1 grazie al passthrough mi fa partire il timer 2 all'inizio del gradino\ntimer_misura.stimulus\t\t= timer_periodo.EVENT_ID \n\n-- Timer 3 controls the pulse width\ntimer_larghezza_impulso.count\t\t\t= 1\ntimer_larghezza_impulso.delay\t\t\t= pulseWidth\n-- il passthrough è false perchè l'interrupt me lo produce alla fine, perchè \ntimer_larghezza_impulso.passthrough\t= false\n--il timer 1 grazie al passthrough mi fa partire il timer 3 all'inizio del gradino\ntimer_larghezza_impulso.stimulus\t\t= timer_periodo.EVENT_ID\n", "gate.source.output\t\t\t\t= gate.OUTPUT_ON\ndrain.source.output\t\t\t\t= drain.OUTPUT_ON\n\n\nfor i=1,numSweep,1 do \n\n-- Configure gate Trigger Model for Sweep\n-- imposto un singolo valore di tensione, costante per tutta la durata della sweep.\n-- quindi quello che ottengo è la sweep di un singolo valore. il risultato è appunto una valore costante\n--in lua a differenza del linguaggio c/c++, il primo elemento di un array ha indice 1, non 0\n\nif source_gate==1 then-----------------------\ngate.trigger.source.listv({livello_gate[i]})\ngate.trigger.source.limiti\t\t= limiti_gate\nelse -------------------------------------------\ngate.trigger.source.listi({livello_gate[i]})\ngate.trigger.source.limitv\t\t= limiti_gate\nend--------------------------------------------\n\ngate.trigger.measure.action\t\t= gate.ASYNC\ngate.trigger.measure.iv(gate.nvbuffer1, gate.nvbuffer2)\n--fine impulso: se voglio una dc sweep, anzichè mandare in idle l'uscita, la tengo costante\ngate.trigger.endpulse.action\t= gate.SOURCE_HOLD\n-- endsweep mi dice cosa fare quando finisce l'operazione sweep\ngate.trigger.endsweep.action\t= gate.SOURCE_HOLD\ngate.trigger.arm.count = 1\ngate.trigger.count\t\t\t\t= 1\n-- arm sweep indica quanto sweep deve fare \ndrain.trigger.arm.stimulus\t\t= 0\n--dico quali timer attivanzo le azioni\n\n--event blender per la partenza\ntrigger.blender[1].orenable = true\ntrigger.blender[1].stimulus[1] = gate.trigger.ARMED_EVENT_ID\ntrigger.blender[1].stimulus[2] = drain.trigger.ARMED_EVENT_ID \n\n--dico quali stimoli/timer attivanzo le azioni\ngate.trigger.source.stimulus = trigger.blender[1].EVENT_ID \ngate.trigger.measure.stimulus\t= trigger.timer[2].EVENT_ID\n--gate.trigger.endpulse.stimulus\t= drain.trigger.SWEEP_COMPLETE_EVENT_ID\ngate.trigger.endpulse.stimulus\t= drain.trigger.IDLE_EVENT_ID\n\ngate.trigger.source.action\t\t= gate.ENABLE\n\n-- Configure drain Trigger Model for Sweep\n\nif source_drain==1 then------------------------\ndrain.trigger.source.linearv(start_drain, stop_drain, numPoints)\ndrain.trigger.source.limiti\t\t= limiti_drain\nelse---------------------------------------------\ndrain.trigger.source.lineari(start_drain, stop_drain, numPoints)\ndrain.trigger.source.limitv\t\t= limiti_drain\nend---------------------------------------------\ndrain.trigger.measure.action\t\t= drain.ENABLE\ndrain.trigger.measure.iv(drain.nvbuffer1, drain.nvbuffer2)\n--fine impulso: se voglio una dc sweep, anzichè mandare in idle l'uscita, la tengo costante\ndrain.trigger.endpulse.action\t= drain.SOURCE_HOLD \n-- endsweep mi dice cosa fare quando finisce l'operazione sweep\ndrain.trigger.endsweep.action\t= drain.SOURCE_HOLD\ndrain.trigger.arm.count = 1\n-- num punti sweep\ndrain.trigger.count\t\t\t\t= numPoints\n-- arm sweep indica quanto sweep deve fare\ndrain.trigger.arm.stimulus\t\t= 0\n--dico quali timer attivanzo le azioni\ndrain.trigger.source.stimulus\t= trigger.timer[1].EVENT_ID\ndrain.trigger.measure.stimulus\t= trigger.timer[2].EVENT_ID\ndrain.trigger.endpulse.stimulus\t= trigger.timer[3].EVENT_ID\ndrain.trigger.source.action\t\t= drain.ENABLE\n--==============================\n-- End Trigger Model Configuration\n\n-- Start the trigger model execution\ngate.trigger.initiate()\ndelay(0.05)\ndrain.trigger.initiate()\n\n-- Wait until the sweep has completed\nwaitcomplete()\n\n\n-- Configure gate Trigger Model for Sweep\n-- imposto un singolo valore di tensione, costante per tutta la durata della sweep.\n-- quindi quello che ottengo è la sweep di un singolo valore. il risultato è appunto una valore costante\nif source_gate==1 then-----------------------\ngate.trigger.source.listv({livello_gate[i]})\ngate.trigger.source.limiti\t\t= limiti_gate\nelse -------------------------------------------\ngate.trigger.source.listi({livello_gate[i]})\ngate.trigger.source.limitv\t\t= limiti_gate\nend--------------------------------------------\ngate.trigger.measure.action\t\t= gate.ASYNC\ngate.trigger.measure.iv(gate.nvbuffer1, gate.nvbuffer2)\n--fine impulso: se voglio una dc sweep, anzichè mandare in idle l'uscita, la tengo costante\ngate.trigger.endpulse.action\t= gate.SOURCE_HOLD\n-- endsweep mi dice cosa fare quando finisce l'operazione sweep\ngate.trigger.endsweep.action\t= gate.SOURCE_HOLD\ngate.trigger.arm.count = 1\ngate.trigger.count\t\t\t\t= 1\n-- arm sweep indica quanto sweep deve fare \ndrain.trigger.arm.stimulus\t\t= 0\n--dico quali timer attivanzo le azioni\n\n--event blender per la partenza\ntrigger.blender[1].orenable = true\ntrigger.blender[1].stimulus[1] = gate.trigger.ARMED_EVENT_ID\ntrigger.blender[1].stimulus[2] = drain.trigger.ARMED_EVENT_ID \n\n--dico quali stimoli/timer attivanzo le azioni\ngate.trigger.source.stimulus = trigger.blender[1].EVENT_ID \ngate.trigger.measure.stimulus\t= trigger.timer[2].EVENT_ID\n--gate.trigger.endpulse.stimulus\t= drain.trigger.SWEEP_COMPLETE_EVENT_ID\ngate.trigger.endpulse.stimulus\t= drain.trigger.IDLE_EVENT_ID\n\n--gate.trigger.source.action\t\t= gate.ENABLE\n\n-- Configure drain Trigger Model for Sweep\n\nif source_drain==1 then------------------------\ndrain.trigger.source.linearv(stop_drain, start_drain, numPoints)\ndrain.trigger.source.limiti\t\t= limiti_drain\nelse---------------------------------------------\ndrain.trigger.source.lineari(stop_drain, start_drain, numPoints)\ndrain.trigger.source.limitv\t\t= limiti_drain\nend---------------------------------------------\ndrain.trigger.measure.action\t\t= drain.ENABLE\ndrain.trigger.measure.iv(drain.nvbuffer1, drain.nvbuffer2)\n--fine impulso: se voglio una dc sweep, anzichè mandare in idle l'uscita, la tengo costante\ndrain.trigger.endpulse.action\t= drain.SOURCE_HOLD \n-- endsweep mi dice cosa fare quando finisce l'operazione sweep\ndrain.trigger.endsweep.action\t= drain.SOURCE_HOLD\ndrain.trigger.arm.count = 1\n-- num punti sweep\ndrain.trigger.count\t\t\t\t= numPoints\n-- arm sweep indica quanto sweep deve fare\ndrain.trigger.arm.stimulus\t\t= 0\n--dico quali timer attivanzo le azioni\ndrain.trigger.source.stimulus\t= trigger.timer[1].EVENT_ID\ndrain.trigger.measure.stimulus\t= trigger.timer[2].EVENT_ID\ndrain.trigger.endpulse.stimulus\t= trigger.timer[3].EVENT_ID\n--drain.trigger.source.action\t\t= drain.ENABLE\n--==============================\n-- End Trigger Model Configuration\n\n-- Start the trigger model execution\ngate.trigger.initiate()\n--delay(0.05)\ndrain.trigger.initiate()\nwaitcomplete()\nend\n\ndrain.source.output\t\t\t\t= drain.OUTPUT_OFF\ndelay(0.05)\ngate.source.output\t\t\t\t= gate.OUTPUT_OFF\n\n--printbuffer(1, numPoints, gate.nvbuffer2.readings)\n--printbuffer(1, numPoints, gate.nvbuffer1.readings)\n--printbuffer(1, numPoints, gate.nvbuffer1.timestamps)\n\n--printbuffer(1, numPoints, drain.nvbuffer2.readings)\n--printbuffer(1, numPoints, drain.nvbuffer1.readings)\n--printbuffer(1, numPoints, drain.nvbuffer1.timestamps)" ("write buffer")) -> (w74:string)
          n15 = Multiply(x=w72, y=2) -> (x*y=w73:i32)
        }
      }
      n16 = Format Into String(format string=w40, w23, w22, w21, w20, w19, w18, w17, w1, w16, w15, w14, w13, w12, w11, w10, w9, w8, w7, w6, w5, w3, w2) -> (resulting string=w49:string)  [unwired: 2 in, 1 out]
      n17 = call <instrlib>:"Create Script.vi"("Auto Run (F: Disable)"=TRUE, "error in (no error)"=w52, "Source Code"=w49, "Script Variable"="myScript", "VISA resource name"=w53) -> ("error out"=w45:errorcluster, "VISA resource name out"=w46:refnum<visa-resource-name>)  [unwired: 5 in]
      n18 = call "lettura_dati.vi"("error in (no error)"=w45, "Source Measure Unit Channel (0: Channel A)"=w42, "End Index (1)"=w38, "VISA resource name"=w46) -> ("error out"=w43:errorcluster, "CORRENTE"=w28:dbl[], "VISA resource name out"=w44:refnum<visa-resource-name>, "TENSIONE"=w35:dbl[], "TEMPI"=w29:dbl[])  [unwired: 3 in]
      n19 = call "lettura_dati.vi"("error in (no error)"=w43, "Source Measure Unit Channel (0: Channel A)"=w41, "End Index (1)"=w38, "VISA resource name"=w44) -> ("error out"=w36:errorcluster, "CORRENTE"=w26:dbl[], "VISA resource name out"=w37:refnum<visa-resource-name>, "TENSIONE"=w34:dbl[], "TEMPI"=w27:dbl[])  [unwired: 3 in]
      n20 = Bundle("VISA resource name out"=w37, "error out"=w36) -> (→"Cluster 2":T2)  [unwired: 1 in]
      n21 = Bundle("CORRENTE"=w28, "TENSIONE"=w35, "TEMPI"=w29, "CORRENTE"=w26, "TENSIONE"=w34, "TEMPI"=w27) -> (→"Cluster 3":T5)  [unwired: 1 in]
    }
  }
